vi "generateSimulatedData.vi"(8 "error in (no error)":errorcluster, 11 "TempSensorSim in":refnum<class "TempSensorSim.lvclass">) -> (0 "error out":errorcluster, 2 "stringRead":string, 3 "TempSensorSim out":refnum<class "TempSensorSim.lvclass">)   [LabVIEW 2013, in "TempSensorSim.lvclass"]
uses:
  TempSensorSim.lvclass
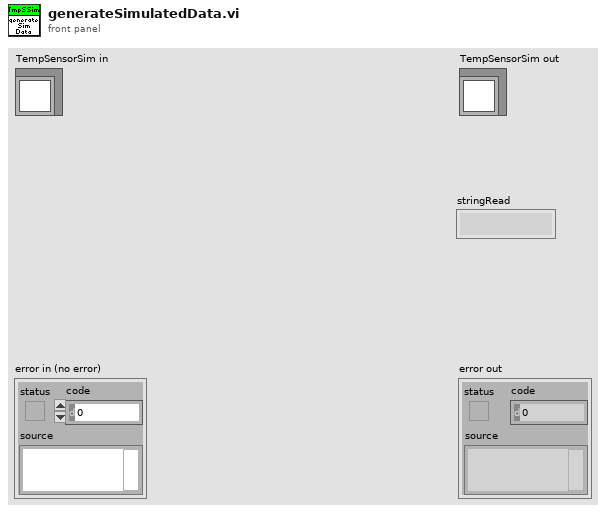
[diagram p1: front panel]
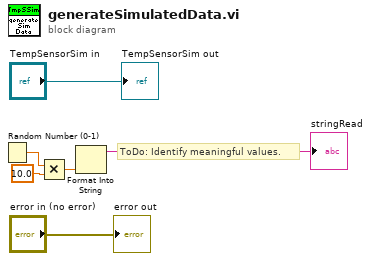
[diagram p0: block diagram]
diagram:
  # "ToDo: Identify meaningful values."
  n1 = Random Number (0-1)() -> (number: 0 to 1=w4:dbl)
  n2 = Multiply(x=w4, y=10.0) -> (x*y=w2:dbl)
  n3 = Format Into String(w2) -> (resulting string=→"stringRead":string)  [unwired: 3 in, 1 out]
  "error out" <- "error in (no error)"
  "TempSensorSim out" <- "TempSensorSim in"
